vi "Delete session file from index.vi"(1 "Workspace path":path, 3 "error in (no error)":errorcluster) -> (7 "Index":T1[](array[typedef]), 10 "error out":errorcluster)   [LabVIEW 2019]
doc: "Removes session file from index of oppened files"
uses:
  Type defs/Opened session file info Type Def.ctl
  Type defs/Opened session file index Type Def.ctl
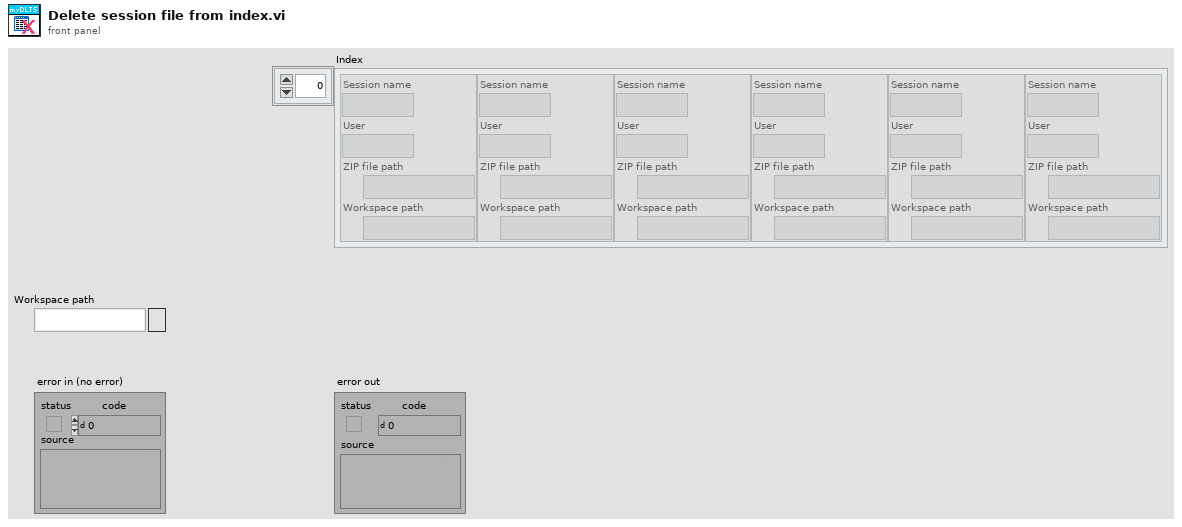
[diagram p1: front panel]
types:
  T1 = typedef "Opened session file info Type Def.ctl" = cluster{"Session name":string, "User":string, "ZIP file path":path, "Workspace path":path}
  T2 = typedef "Opened session file index Type Def.ctl" = cluster{"File":T1[]}
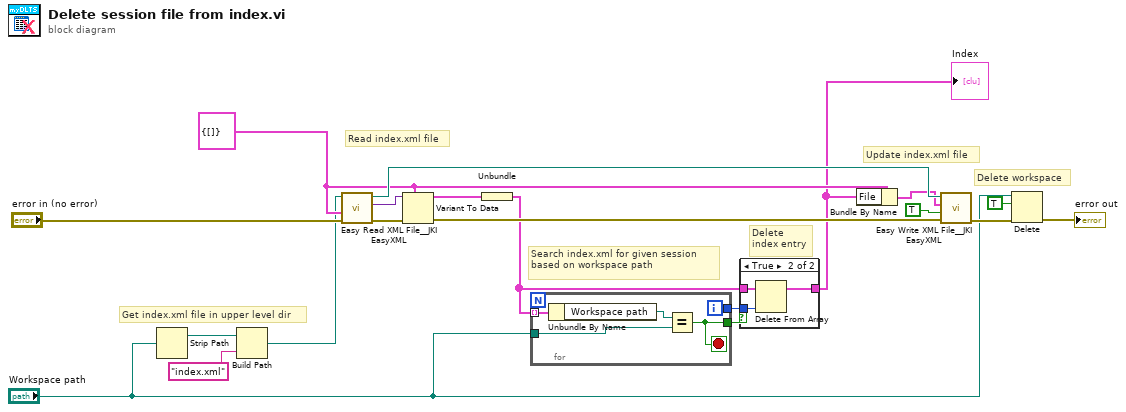
[diagram p0: block diagram]
diagram:
  w13 = T2 {"File"=[]} ("Index")
  # "Delete workspace"
  # "Update index.xml file"
  # "Delete index entry"
  # "Search index.xml for given session based on workspace path"
  # "Read index.xml file"
  # "Get index.xml file in upper level dir"
  n1 = Strip Path(path="Workspace path") -> (stripped path=w6:path)  [unwired: 1 out]
  n2 = Build Path(base path=w6, name or relative path="index.xml") -> (appended path=w7:path)
  n3 = call <vilib>:"Easy Read XML File__JKI EasyXML.vi"("error in (no error)"="error in (no error)", "LabVIEW Data (Type)"=w13, "XML File Path"=w7) -> ("error out"=w20:errorcluster, "LabVIEW Data"=w17:variant, "XML File Path (duplicate)"=w16:path)  [unwired: 6 in]
  n4 = Variant To Data(error in=w20, type=w13, Variant=w17) -> (data=w15:T2, error out=w19:errorcluster)
  n5 = Unbundle(w15) -> ("File"=w9:T1[])
  n6 = for {
    tunnel: w9 -> [w25] mode=indexing
    tunnel: "Workspace path" -> [w23]
    tunnel: [w22] -> w11
    tunnel: [w21] -> w10
    i -> [w21]
    stop <- w22 stop-if-true
    n7 = Unbundle By Name(w25) -> ("Workspace path"=w24:path)
    n8 = Equal?(x=w24, y=w23) -> (x = y?=w22:bool)
  }
  n9 = case shown="True" w11 {
    tunnel: w10 -> [_ w29]
    tunnel: w9 -> [w26 w28]
    tunnel: [w26 w27] -> w8
    frame False {
    }
    frame True {
      n10 = Delete From Array(array=w28, index=w29) -> (array with subset deleted=w27:T1[])  [unwired: 1 in, 1 out]
    }
  }
  "Index" <- w8
  n11 = Bundle By Name(cluster=w13, "File"=w8) -> (w12:T2)
  n12 = call <vilib>:"Easy Write XML File__JKI EasyXML.vi"("error in (no error)"=w19, "Overwrite File? (false)"=TRUE, "LabVIEW Data"=w12, "XML File Path"=w16) -> ("error out"=w4:errorcluster)  [unwired: 6 in, 1 out]
  n13 = Delete(path (use dialog)="Workspace path", entire hierarchy (F)=TRUE, error in=w4) -> (error out=→"error out":errorcluster)  [unwired: 2 in, 2 out]
